vi "ActionVIOnCompile.vi"(8 "error in (no error)":errorcluster, 11 "Device Item Ref in":T1 format="%.0x") -> (0 "error out":errorcluster)   [LabVIEW 2016, in "NI Synchronization System Explorer.lvlib"]
uses:
  NI Synchronization System Explorer.lvlib
  <vilib>/NI Veristand/Custom Device API/Custom Device Item Ref.ctl
  <vilib>/NI Veristand/Custom Device API/Set Item Property (Boolean).vi
  <vilib>/NI Veristand/Custom Device API/Custom Device API.lvlib
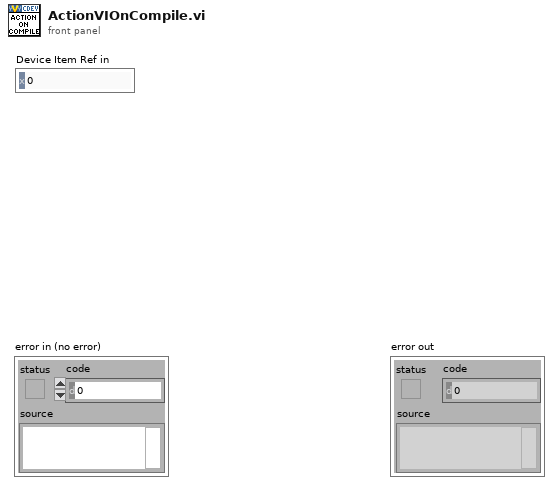
[diagram p1: front panel]
types:
  T1 = typedef "Custom Device API.lvlib/Custom Device Item Ref.ctl" = u64
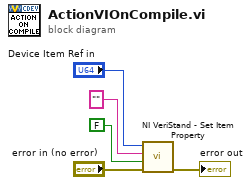
[diagram p0: block diagram]
diagram:
  n1 = call-poly <vilib>:"NI VeriStand - Set Item Property.vi"("error in (no error)"="error in (no error)", "Value"=FALSE, "Property Name"="", "Item Ref in"="Device Item Ref in") -> ("error out"=→"error out":errorcluster)  [unwired: 5 in, 2 out]
